vi "InstaCoverage Time Measurement Runner.vi"() -> ()   [LabVIEW 2018]
uses:
  Common Support/Test File Path--cluster.ctl
  Common Support/Common Support.lvlib
panel:
  out "Executed Test Count":i32
  in  "Calculate Temperature Change":bool=TRUE
  in  "Thermal Chamber Response Simulator_Init":bool=TRUE
  in  "Get Chamber Status":bool=TRUE
  in  "GUI Interlock Tester":bool=TRUE
  in  "Convert Shutdown Furnace to Heater State Enum":bool=TRUE
  in  "All Test":bool
  out "ICov In Progress":bool
  out "ICov Testing time (seconds)":dbl
  out "ICov Results":enum16{"PASSED", "FAILED", "ERROR"}[](array[ring])
  in  "Action Update Heater State":bool=TRUE
  in  "Action Update Set Point":bool=TRUE
  in  "Action Update Ramp Rate":bool=TRUE
  in  "Multiplier of runs":i32=10
  # "If \"All Test\" is true, then all of selected and unselected tests \nbelow will be executed and each test will be executed only \nonce independently of \"Multiplier of runs\"."
  # "ICov"
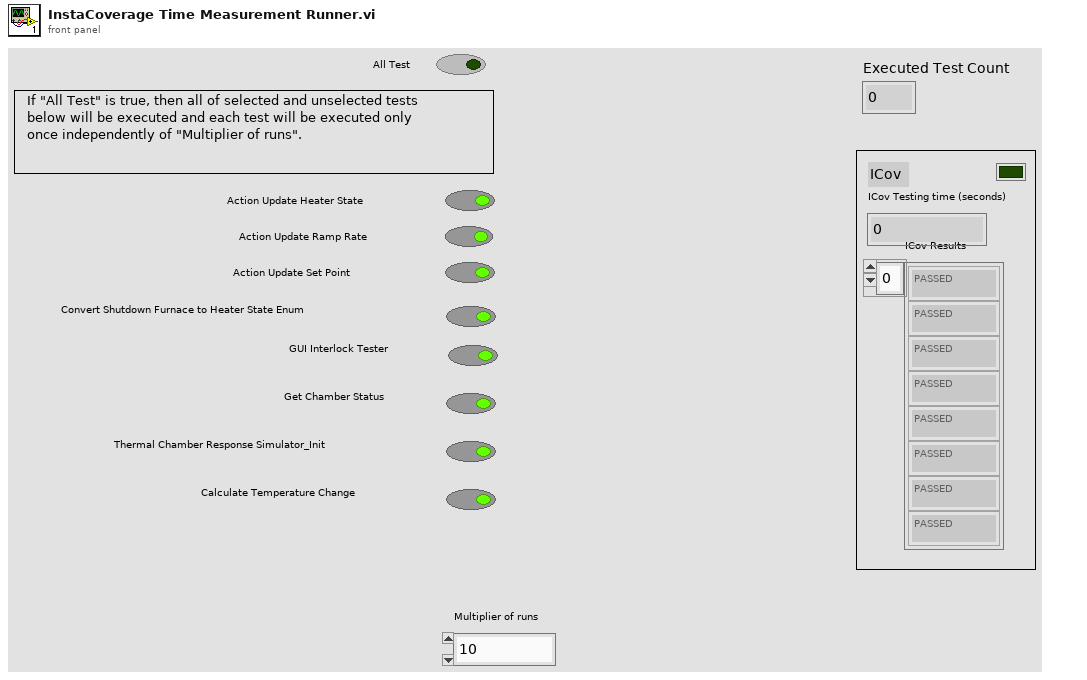
[diagram p1: front panel]
types:
  T1 = typedef "Common Support.lvlib/Test File Path--cluster.ctl" = cluster{"Folder Name":string, "Test File Name":string}
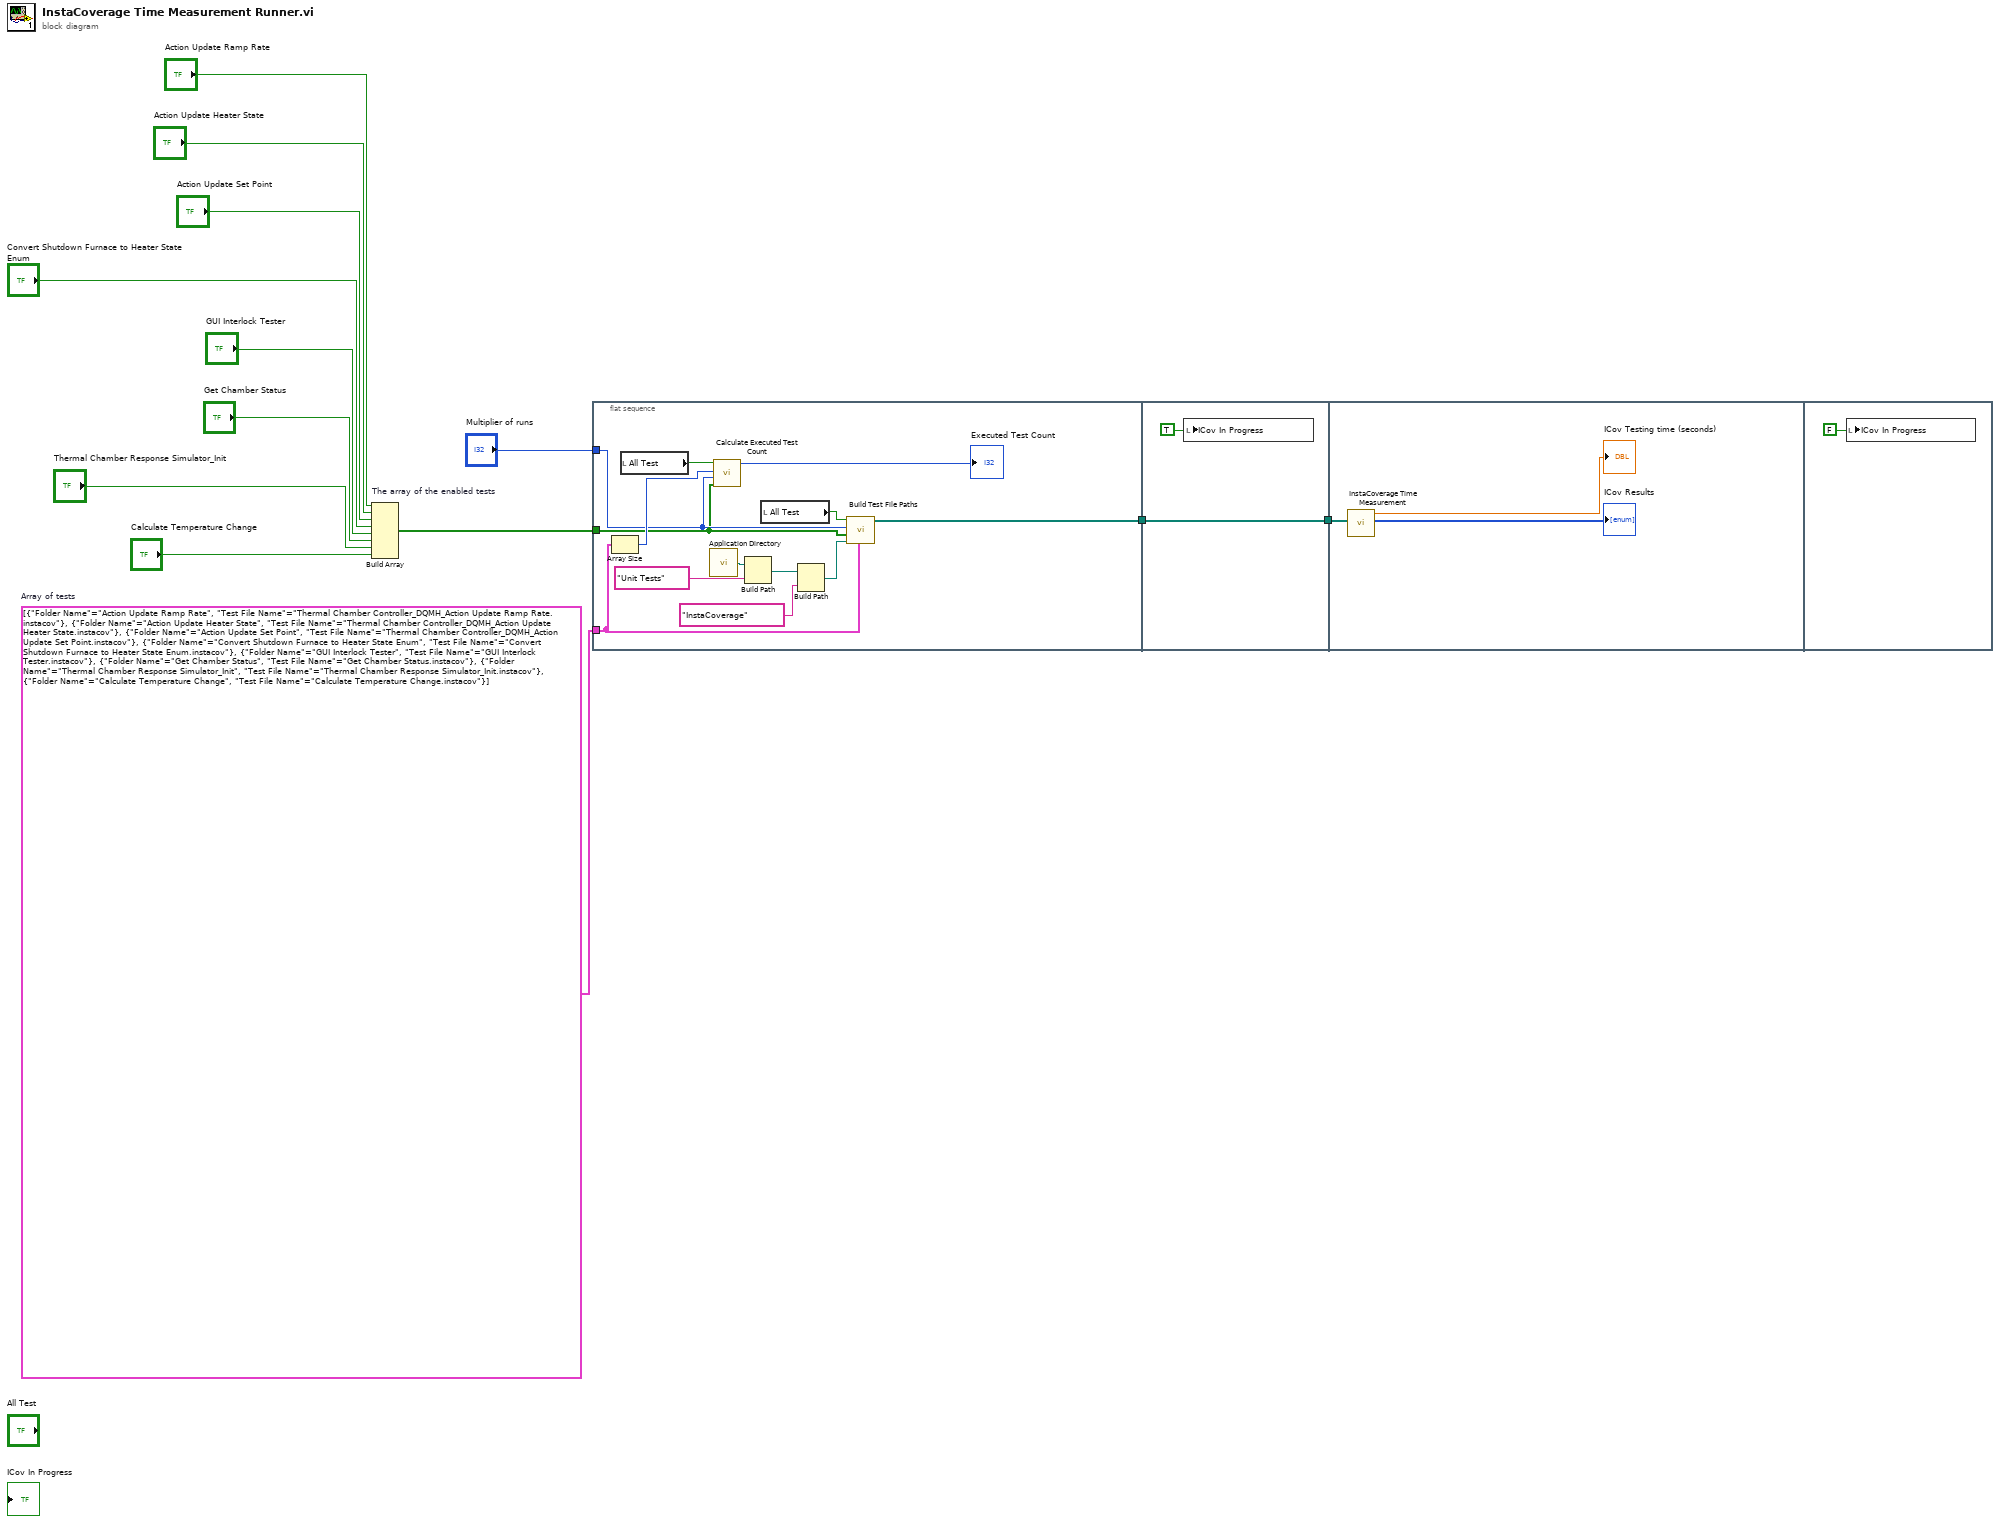
[diagram p0: block diagram]
diagram:
  w13 = T1[] [{"Folder Name"="Action Update Ramp Rate", "Test File Name"="Thermal Chamber Controller_DQMH_Action Update Ramp Rate.instacov"}, {"Folder Name"="Action Update Heater State", "Test File Name"="Thermal Chamber Controller_DQMH_Action Update Heater State.instacov"}, {"Folder Name"="Action Update Set Point", "Test File Name"="Thermal Chamber Controller_DQMH_Action Update Set Point.instacov"}, {"Folder Name"="Convert Shutdown Furnace to Heater State Enum", "Test File Name"="Convert Shutdown Furnace to Heater State Enum.instacov"}, {"Folder Name"="GUI Interlock Tester", "Test File Name"="GUI Interlock Tester.instacov"}, {"Folder Name"="Get Chamber Status", "Test File Name"="Get Chamber Status.instacov"}, {"Folder Name"="Thermal Chamber Response Simulator_Init", "Test File Name"="Thermal Chamber Response Simulator_Init.instacov"}, {"Folder Name"="Calculate Temperature Change", "Test File Name"="Calculate Temperature Change.instacov"}]  # Array of tests
  n1 = Build Array "The array of the enabled tests"("Action Update Ramp Rate", "Action Update Heater State", "Action Update Set Point", "Convert Shutdown Furnace to Heater State Enum", "GUI Interlock Tester", "Get Chamber Status", "Thermal Chamber Response Simulator_Init", "Calculate Temperature Change") -> (w6:bool[])
  n2 = flat-sequence {
    tunnel: w13 -> [w18]
    tunnel: "Multiplier of runs" -> [w16]
    tunnel: [w22] -> w11
    tunnel: w6 -> [w15]
    tunnel: w11 -> [w27]
    tunnel: [w27] -> w10
    tunnel: w10 -> [w29]
    frame #0 {
      n3 = Array Size(array=w18) -> (size(s)=w17:i32)
      n4 = local read "All Test"() -> (w19:bool)
      n5 = call <vilib>:"Application Directory.vi"() -> ("Application Directory"=w26:path)
      n6 = call "Calculate Executed Test Count.vi"("Test Selector Array"=w15, "Multiplier of Runs"=w16, "All Test Count"=w17, "Run All Tests"=w19) -> ("Executed Test Count"=→"Executed Test Count":i32)  [unwired: 7 in]
      n7 = Build Path(base path=w26, name or relative path="Unit Tests") -> (appended path=w23:path)
      n8 = local read "All Test"() -> (w21:bool)
      n9 = Build Path(base path=w23, name or relative path="InstaCoverage") -> (appended path=w20:path)
      n10 = call "Build Test File Paths.vi"("Test Files"=w18, "Tests Folder Path"=w20, "Runnable Test Selector"=w15, "Multiplier of runs"=w16, "Run All"=w21) -> ("Test File Paths to Execute"=w22:path[])  [unwired: 6 in]
    }
    frame #1 {
      n11 = local write "ICov In Progress"(TRUE ("ICov In Progress")) -> ()
    }
    frame #2 {
      n12 = call "InstaCoverage Time Measurement.vi"("test file paths"=w29) -> ("ICov Results"=→"ICov Results":enum16{"PASSED", "FAILED", "ERROR"}[], "ICov Testing time (seconds)"=→"ICov Testing time (seconds)":dbl)  [unwired: 9 in]
    }
    frame #3 {
      n13 = local write "ICov In Progress"(FALSE ("ICov In Progress")) -> ()
    }
  }
